vi "to json str.vi"(8 "error in (no error)":errorcluster, 11 "Request in":refnum<class "Request.lvclass">) -> (0 "error out":errorcluster, 2 "request str":string, 3 "Request out":refnum<class "Request.lvclass">)   [LabVIEW 2018, in "Request.lvclass"]
uses:
  Request.lvclass
  Request.lvclass/Request.ctl
  Command/Command.lvclass/Command.ctl
  Command/Command.lvclass
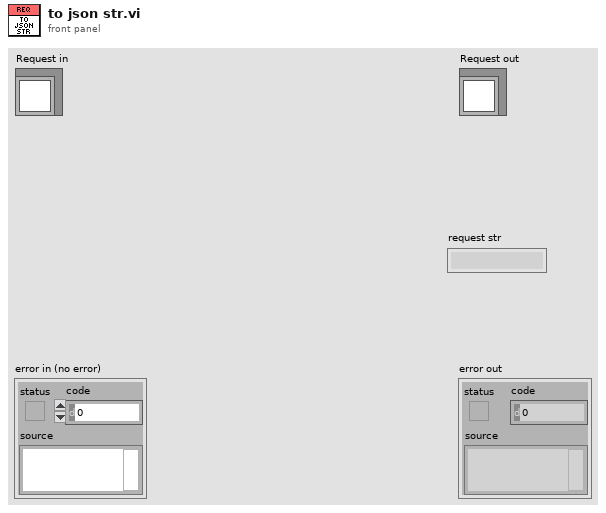
[diagram p1: front panel]
types:
  T1 = cluster{"device":string, "action":string, "parameter":string}
  T2 = cluster{"command":cluster{"device":string, "action":string, "parameter":string}, "timestamp":string, "broker":string}
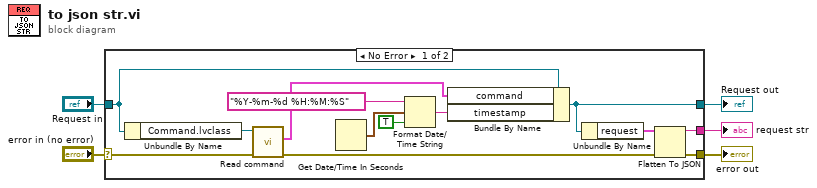
[diagram p0: block diagram]
diagram:
  n1 = case shown="No Error" "error in (no error)" {
    selector: "error in (no error)" -> [w15 w20]
    tunnel: [w9 w20] -> w4
    tunnel: [w12 w19] -> w2
    tunnel: "Request in" -> [w18 w19]
    tunnel: [w10 _] -> w1
    frame No Error {
      n2 = Unbundle By Name(w18) -> ("Command.lvclass"=w17:refnum<class "Command.lvclass">)
      n3 = call "Read command.vi"("error in (no error)"=w15, "Command in"=w17) -> ("error out"=w8:errorcluster, "command"=w16:T1)  [unwired: 7 in, 1 out]
      n4 = Get Date/Time In Seconds() -> (seconds since 1Jan1904=w14:timestamp)
      n5 = Format Date/Time String(time format string (%c)="%Y-%m-%d %H:%M:%S", seconds (now)=w14, UTC format=TRUE) -> (date/time string=w13:string)
      n6 = Bundle By Name(cluster=w18, "command"=w16, "timestamp"=w13) -> (w12:refnum<class "Request.lvclass">)
      n7 = Unbundle By Name(w12) -> ("request"=w11:T2)
      n8 = Flatten To JSON(anything=w11, error in (no error)=w8) -> (JSON string=w10:string, 11:w9:errorcluster)  [unwired: 1 in]
    }
    frame Error {
    }
  }
  "error out" <- w4
  "Request out" <- w2
  "request str" <- w1
